vi "golpi_mpc_check_state.vi"(8 "error in":errorcluster, 11 "golpi session ref":T3) -> (0 "error out":errorcluster, 1 "GOLPI busy?":bool, 2 "GOLPI ready?":bool, 3 "golpi session ref out":T3, 4 "GOLPI running?":bool, 5 "GOLPI ref":T1={"pipe handle"={"lv_proc.dll file path"=path "", "process instance handle"=[], "debug mode"=FALSE, "debug data"=[]}, "fast read timeout [ms]"=500, "fast read settle time [ms]"=10, "fast read to multiple [ms]"=1, "max elements per input line"=100, "slow read timeout [ms]"=5000, "stdin double format specifier"="%_16e", "max elements per stdout output column"=100, "console mode bitstream"=FALSE, "bitstream first read timeout [ms]"=1000, "bitstream read timeout [ms]"=50, "struct transfer possible"=FALSE, "matlab mode"=FALSE})   [LabVIEW 2020, in "GOLPI Multi Process.lvlib"]
doc: "Call this to check if access to GOLPI is available or busy."
uses:
  GOLPI Multi Process.lvlib
  golpi_session_ref.ctl
  golpi_session.ctl
  GOLPI reference Type Def.ctl
  Pipe Handle.ctl
  GOLPI library.lvlib
  LV Process library.lvlib
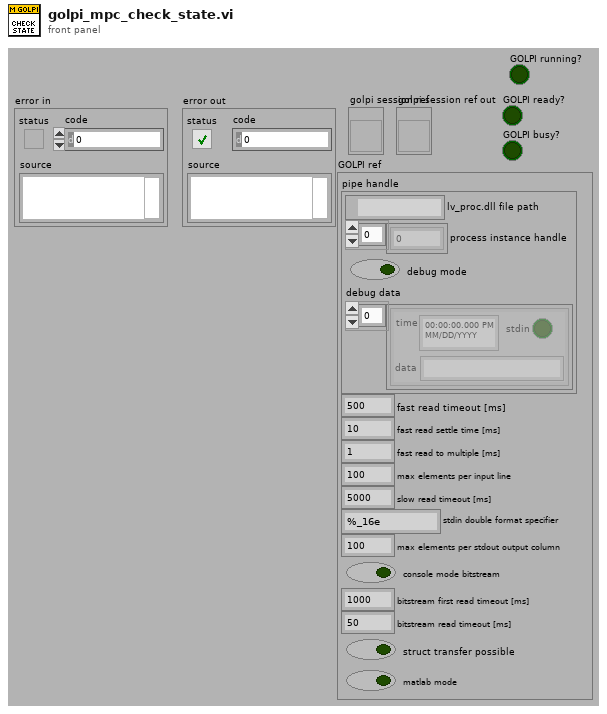
[diagram p1: front panel]
types:
  T1 = typedef "GOLPI library.lvlib/GOLPI reference Type Def.ctl" = cluster{"pipe handle":T2, "fast read timeout [ms]":u32, "fast read settle time [ms]":u32, "fast read to multiple [ms]":u32, "max elements per input line":u32, "slow read timeout [ms]":u32, "stdin double format specifier":string, "max elements per stdout output column":u32, "console mode bitstream":bool, "bitstream first read timeout [ms]":u32, "bitstream read timeout [ms]":u32, "struct transfer possible":bool, "matlab mode":bool}
  T2 = typedef "LV Process library.lvlib/Pipe Handle.ctl" = cluster{"lv_proc.dll file path":path, "process instance handle":u32[], "debug mode":bool, "debug data":cluster{"time":timestamp, "stdin":bool, "data":string}[]}
  T3 = typedef "GOLPI Multi Process.lvlib/golpi_session_ref.ctl" = refnum<vi>
  T4 = typedef "GOLPI Multi Process.lvlib/golpi_session.ctl" = cluster{"GOLPI ref":T1, "idn str":string, "octave path":path, "work path":path, "start timeout [ms]":u32, "clr cache":bool, "console":bool, "binary":bool, "semaphore":T5, "initial command":string, "exit command":string, "matlab":bool, "pkg list":string[]}
  T5 = typedef "Semaphore RefNum" = refnum<k1>
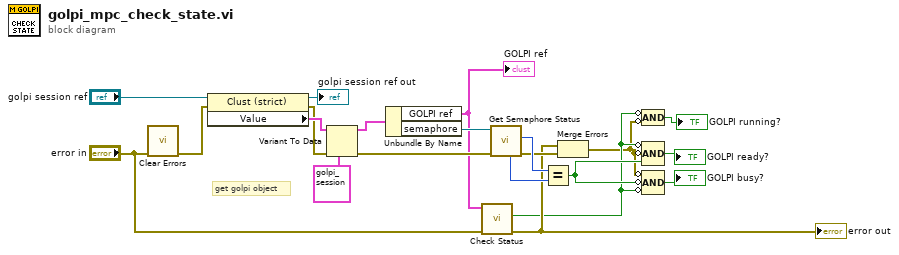
[diagram p0: block diagram]
diagram:
  # "get golpi object"
  n1 = call <vilib>:"Clear Errors.vi"("error in (no error)"="error in") -> ("error out"=w17:errorcluster)  [unwired: 5 in, 1 out]
  n2 = property class="Clust (strict)"(reference="golpi session ref", error in=w17) -> (reference out=→"golpi session ref out":T3, error out=w18:errorcluster, "Value"=w21:T4)
  n3 = Variant To Data(error in=w18, type=T4 {"GOLPI ref"={"pipe handle"={"lv_proc.dll file path"=path "", "process instance handle"=[], "debug mode"=FALSE, "debug data"=[]}, "fast read timeout [ms]"=0, "fast read settle time [ms]"=0, "fast read to multiple [ms]"=0, "max elements per input line"=0, "slow read timeout [ms]"=0, "stdin double format specifier"="", "max elements per stdout output column"=0, "console mode bitstream"=FALSE, "bitstream first read timeout [ms]"=0, "bitstream read timeout [ms]"=0, "struct transfer possible"=FALSE, "matlab mode"=FALSE}, "idn str"="", "octave path"=path "C:/Octave364/Octave3.6.4_gcc4.6.2/bin", "work path"=path "", "start timeout [ms]"=0, "clr cache"=FALSE, "console"=FALSE, "binary"=FALSE, "semaphore"=refnum, "initial command"="", "exit command"="", "matlab"=FALSE, "pkg list"=[]} ("golpi session"), Variant=w21) -> (data=w19:T4, error out=w15:errorcluster)
  n4 = Unbundle By Name(w19) -> ("GOLPI ref"=w7:T1, "semaphore"=w14:T5)
  "GOLPI ref" <- w7
  n5 = call "Check Status.vi"("error in"="error in", "GOLPI ref. in"=w7) -> ("error out"=w4:errorcluster, "exited?"=w3:bool)  [unwired: 7 in, 1 out]
  "error out" <- w4
  n6 = call <vilib>:"Get Semaphore Status.vi"("error in (no error)"=w15, "semaphore"=w14) -> ("error out"=w5:errorcluster, "# available"=w13:i32, "size"=w12:i32)  [unwired: 4 in, 3 out]
  n7 = Equal?(x=w13, y=w12) -> (x = y?=w10:bool)
  n8 = Merge Errors(w4, w5) -> (w2:errorcluster)
  n9 = Compound Arithmetic op=AND(invert w3, invert w2) -> (→"GOLPI running?":bool)
  n10 = Compound Arithmetic op=AND(invert w3, invert w2, w10) -> (→"GOLPI ready?":bool)
  n11 = Compound Arithmetic op=AND(invert w2, invert w10, invert w3) -> (→"GOLPI busy?":bool)
